vi "bats.parser.ip.vi"() -> ()   [LabVIEW 2022 SP3]
uses:
  data.ctl
  <vilib>/Platform/TimedLoop/XDataNode/timing_clust.ctl
  <vilib>/Platform/TimedLoop/XDataNode/nitl_modes.ctl
  <vilib>/Platform/TimedLoop/XDataNode/wakeup.ctl
  <vilib>/rvi/Emulation/niFpgaSctlEmulationGetInTimedLoop.vi
  <vilib>/rvi/Emulation/niFpgaEmulationReportErrorSimple.vi
  <vilib>/rvi/Emulation/niFpgaGetClockAttributes.vi
  <vilib>/rvi/Emulation/niFpgaCriticalErrorInLSC.vi
  <vilib>/rvi/Emulation/niFpgaEmulationIsFPGAContextNoSignature.vi
  <vilib>/rvi/errors/niFpgaSetErrorForExecOnDevCompSimple.vi
  <vilib>/rvi/eio/common/nirviEmuReportErrorAndStop.vi
  <vilib>/rvi/DataTransferAndStorage/Container/Common/niFpgaContainerGetUniqueNameForEmu.vi
  <vilib>/rvi/FIFO/Fifo_Resource/nirvififoEmulationSetSize.vi
  <vilib>/rvi/FIFO/Fifo_Resource/nirviFifoEmulationQueueMgr.vi
  <instcachedir>/0/nirviFifoEmulationQueueMgr_E5CAEC123FF24DC58D834DCA3CDAA9B5.lvgen/nirviFifoEmulationQueueMgr_E5CAEC123FF24DC58D834DCA3CDAA9B5_000.vi
  <vilib>/Utility/error.llb/Clear Errors.vi
  <vilib>/rvi/FIFO/Fifo_Resource/nirvififoEmulationCreateLock.vi
  <vilib>/rvi/Emulation/niFpgaProcessEmulError.vi
  <vilib>/rvi/FIFO/Fifo_Resource/nirvififoEmulationObtainLock.vi
  <vilib>/rvi/FIFO/Fifo_Resource/nirvififoEmulationReleaseLock.vi
  <vilib>/rvi/occurrence/nirviWaitOnOccurrenceBase.vi
  <vilib>/rvi/errors/nirviReportUnexpectedCaseInternalError.vi
  <vilib>/rvi/errors/nirviReportUnexpectedCaseInternalError (U32).vi
  <instcachedir>/0/nirviFifoEmulationQueueMgr_E5CAEC123FF24DC58D834DCA3CDAA9B5.lvgen/nirviFifoEmulationQueueMgr_E5CAEC123FF24DC58D834DCA3CDAA9B5_026.vi
  <vilib>/Platform/TimedLoop/XDataNode/XDataNode.xnode
  <vilib>/rvi/DataTransferAndStorage/Container/XNode/niFpgaContainer.xnode
  <vilib>/rvi/FIFO/Fifo_Resource/nirvififoEmulationRead.vi
  <vilib>/Platform/TimedLoop/XDataNode/XDNodeRunTimeDep.lvlib
panel:
  out "Nanoseconds (U64)":u64
  out "Seconds (U64)":u64
  out "Remaining Quantity (U32)":u32
  out "OrderBook Command.Type":T1(ring)
  out "Debug.Valid":bool
  out "Debug.Element":u64
  in  "Ready.For.Debug":bool
  in  "data":T2={"enabled"=[FALSE, FALSE, FALSE, FALSE, FALSE, FALSE, FALSE, FALSE], "byte"=[0, 0, 0, 0, 0, 0, 0, 0]} {"byte" format="%.0x"}
  out "OrderBook.Command.Valid":bool
  out "Canceled Quantity (U32)":u32
  out "Executed Quantity (U32)":u32
  out "Price (U64)":u64
  out "Symbol (U64)":u64
  out "Quantity (U32)":u32
  out "Order Id (U64)":u64
  out "Side (U8)":u8
  in  "Ready.for.OrderBook.Command":bool
  out "Ready.for.Udp.Input":bool
  in  "data.valid":bool
  in  "reset":bool
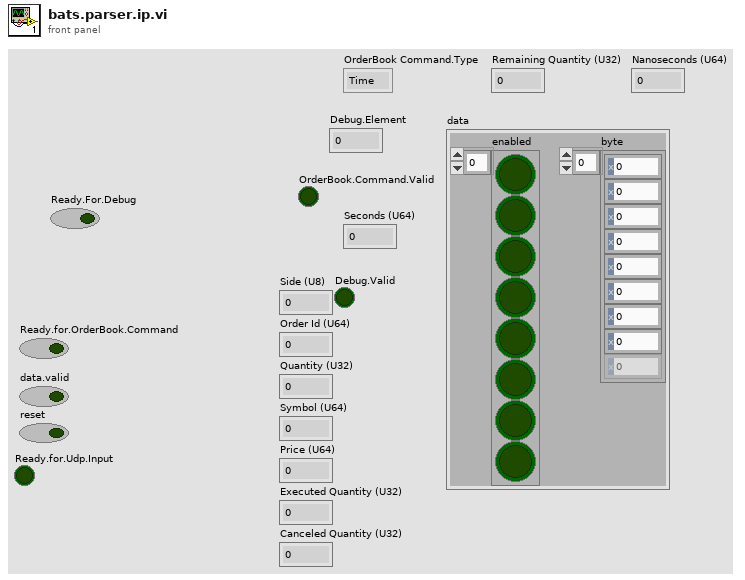
[diagram p1: front panel]
types:
  T1 = enum8{"Time", "AddOrder", "OrderExecuted", "OrderExecutedAtPrice", "ReduceSize", "ModifyOrder", "DeleteOrder", "Get.Everything", "Get.All.Orders", "Get.Top"}
  T2 = typedef "data.ctl" = cluster{"enabled":bool[], "byte":u8[]}
  T3 = typedef "XDNodeRunTimeDep.lvlib/timing_clust.ctl" = cluster{"Expected End [f-1]":u64, "Actual End [f-1]":u64, "Finished Late? [f-1]":bool, "Expected End [i-1]":u64, "Actual End [i-1]":u64, "Finished Late? [i-1]":bool, "Expected Start [i]":u64, "Actual Start [i]":u64, "Expected Start [f]":u64, "Actual Start [f]":u64, "Source Name":string, "Structure Name":string, "Period":i64, "Deadline":i64, "Offset":i64, "Start":i64, "Priority":i32, "Timeout":i32, "Mode":T4, "Wakeup Reason":T5, "Error":errorcluster, "Source Type":string, "Secondary Source Type":string, "Global End Time":u64, "Global Start Time":u64, "Frame Duration":u64, "Iteration Duration":u64, "Assigned CPU":i32, "I/O Scan Engine Mode":u32}
  T4 = typedef "XDNodeRunTimeDep.lvlib/nitl_modes.ctl" = enum32{"No Change", "Process missed periods, maintain original phase", "Discard missed periods, maintain original phase", "Process missed periods, ignore original phase", "Discard missed periods, ignore original phase"}
  T5 = typedef "XDNodeRunTimeDep.lvlib/wakeup.ctl" = enum32{"Normal", "Aborted", "Asynchronous wakeup", "Timing source error", "Timed loop error", "Timeout"}
  T6 = cluster{"type":enum8{"Time", "AddOrder", "OrderExecuted", "OrderExecutedAtPrice", "ReduceSize", "ModifyOrder", "DeleteOrder", "Get.Everything", "Get.All.Orders", "Get.Top"}, "side":u8, "orderId ":u64, "quantity":u32, "symbol":u64, "price":u64, "executed.qty":u32, "canceled.qty":u32, "remaining.qty":u32, "seconds":u64, "nanoseconds":u64, "Add":bool, "Edit":bool, "Remove":bool}
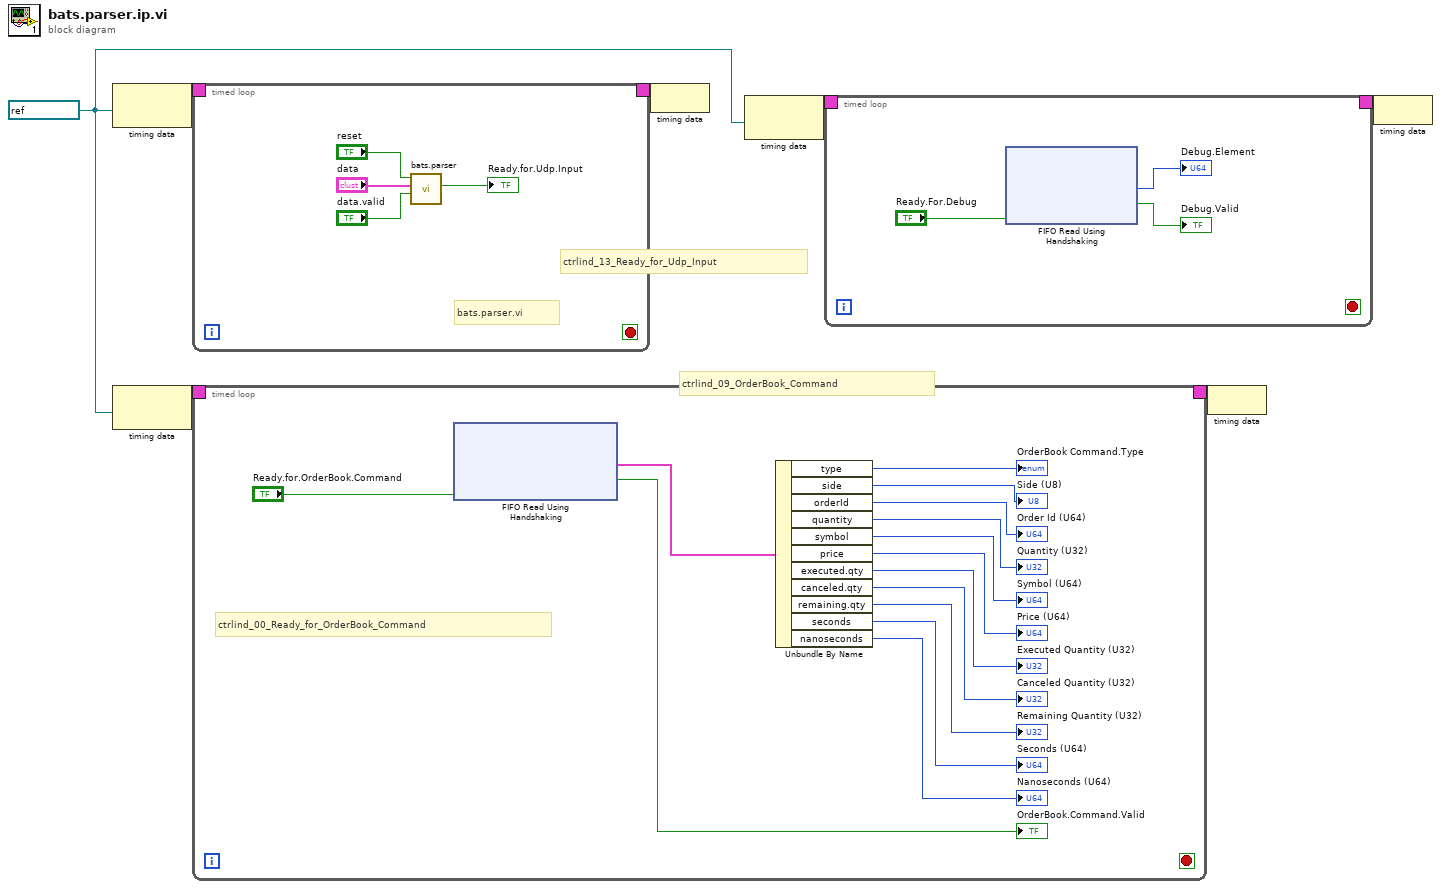
[diagram p0: block diagram]
diagram:
  w1 = refnum<k21> "160MHz" ("Source Name")
  # "ctrlind_09_OrderBook_Command"
  # "ctrlind_13_Ready_for_Udp_Input"
  n1 = node-c288(w1) -> (w7:T3)
  n2 = node-c288(w1) -> (w5:T3)
  n3 = timed-loop {
    timing: w7 -> [_]
    timing-out: [_] -> w6
    stop <- _ stop-if-true
    # "bats.parser.vi"
    n4 = call "bats.parser.vi"("data.valid"="data.valid", "data"="data", "reset"="reset") -> ("Ready.for.Udp.Input"=→"Ready.for.Udp.Input":bool)  [unwired: 8 in]
  }
  n5 = timed-loop {
    timing: w5 -> [_]
    timing-out: [_] -> w4
    stop <- _ stop-if-true
    # "ctrlind_00_Ready_for_OrderBook_Command"
    n6 = xnode ("FIFO Read Using Handshaking")("Ready for Output"="Ready.for.OrderBook.Command") -> ("Element"=w20:T6, "Output Valid"=→"OrderBook.Command.Valid":bool)  [unwired: 1 in, 1 out]
    n7 = Unbundle By Name(w20) -> ("type"=→"OrderBook Command.Type":T1, "side"=→"Side (U8)":u8, "orderId"=→"Order Id (U64)":u64, "quantity"=→"Quantity (U32)":u32, "symbol"=→"Symbol (U64)":u64, "price"=→"Price (U64)":u64, "executed.qty"=→"Executed Quantity (U32)":u32, "canceled.qty"=→"Canceled Quantity (U32)":u32, "remaining.qty"=→"Remaining Quantity (U32)":u32, "seconds"=→"Seconds (U64)":u64, "nanoseconds"=→"Nanoseconds (U64)":u64)
  }
  n8 = node-c288(w6) -> ()
  n9 = node-c288(w1) -> (w3:T3)
  n10 = timed-loop {
    timing: w3 -> [_]
    timing-out: [_] -> w2
    stop <- _ stop-if-true
    n11 = xnode ("FIFO Read Using Handshaking")("Ready for Output"="Ready.For.Debug") -> ("Element"=→"Debug.Element":u64, "Output Valid"=→"Debug.Valid":bool)  [unwired: 1 in, 1 out]
  }
  n12 = node-c288(w4) -> ()
  n13 = node-c288(w2) -> ()
